vi "Ref Time series save images.vi"(8 "error in (no error)":errorcluster, 9 "Ch1-Green-REF":i16[][](graph), 10 "Ch0-Red-REF":i16[][](graph), 11 "Logging queue element":T2={"Imaging Protocol"=enum."Live Imaging", "Number of Trials"=0, "Frame Size"=512, "# Averaged frames"=0, "Dwell time (us)"=0.0, "Index of Z-plane"=0, "Timelapse?"=FALSE, "Logging process is active"=FALSE, "Speed logging enabled"=FALSE, "tdms file ref"=refnum, "path"=path "", "Trial Number"=0, "Expected # points acquired"=FALSE, "Manually stopped"=FALSE, "Last trial"=FALSE, "Ch0 data"=[], "Ch1 data"=[], "Ref Data"=[], "Ref Frame Time"=[], "Image Time"=[], "Continuous Time"=[], "Ref X Length"=0, "Ref Y Length"=0, "# Ref Averaged frames"=0, "Ref Dwell time (us)"=0.0, "Points acquired"={"Ch0 last trial"=0, "Ch1 last trial"=0, "All trials"=0}, "HW Timings File"=refnum} {"Ref Dwell time (us)" format="%#.6g"; "Frame Size" items=["100X100"=100, "128X128"=128, "200X200"=200, "256X256"=256, "512X512"=512, "1024x1024"=1024, "2048x2048"=2048]; "Dwell time (us)" format="%#.6g"}) -> (0 "error":errorcluster)   [LabVIEW 2020]
uses:
  Typedefs/Logging queue element.ctl
  Typedefs/Imaging Protocols enum.ctl
  Typedefs/Frame Size.ctl
  Typedefs/Acquired points count.ctl
  Typedefs/Channel Selector.ctl
  Typedefs/Read Write Enum.ctl
  Global Variables/General Globals.vi
panel:
  out "Imaging Protocol":T1
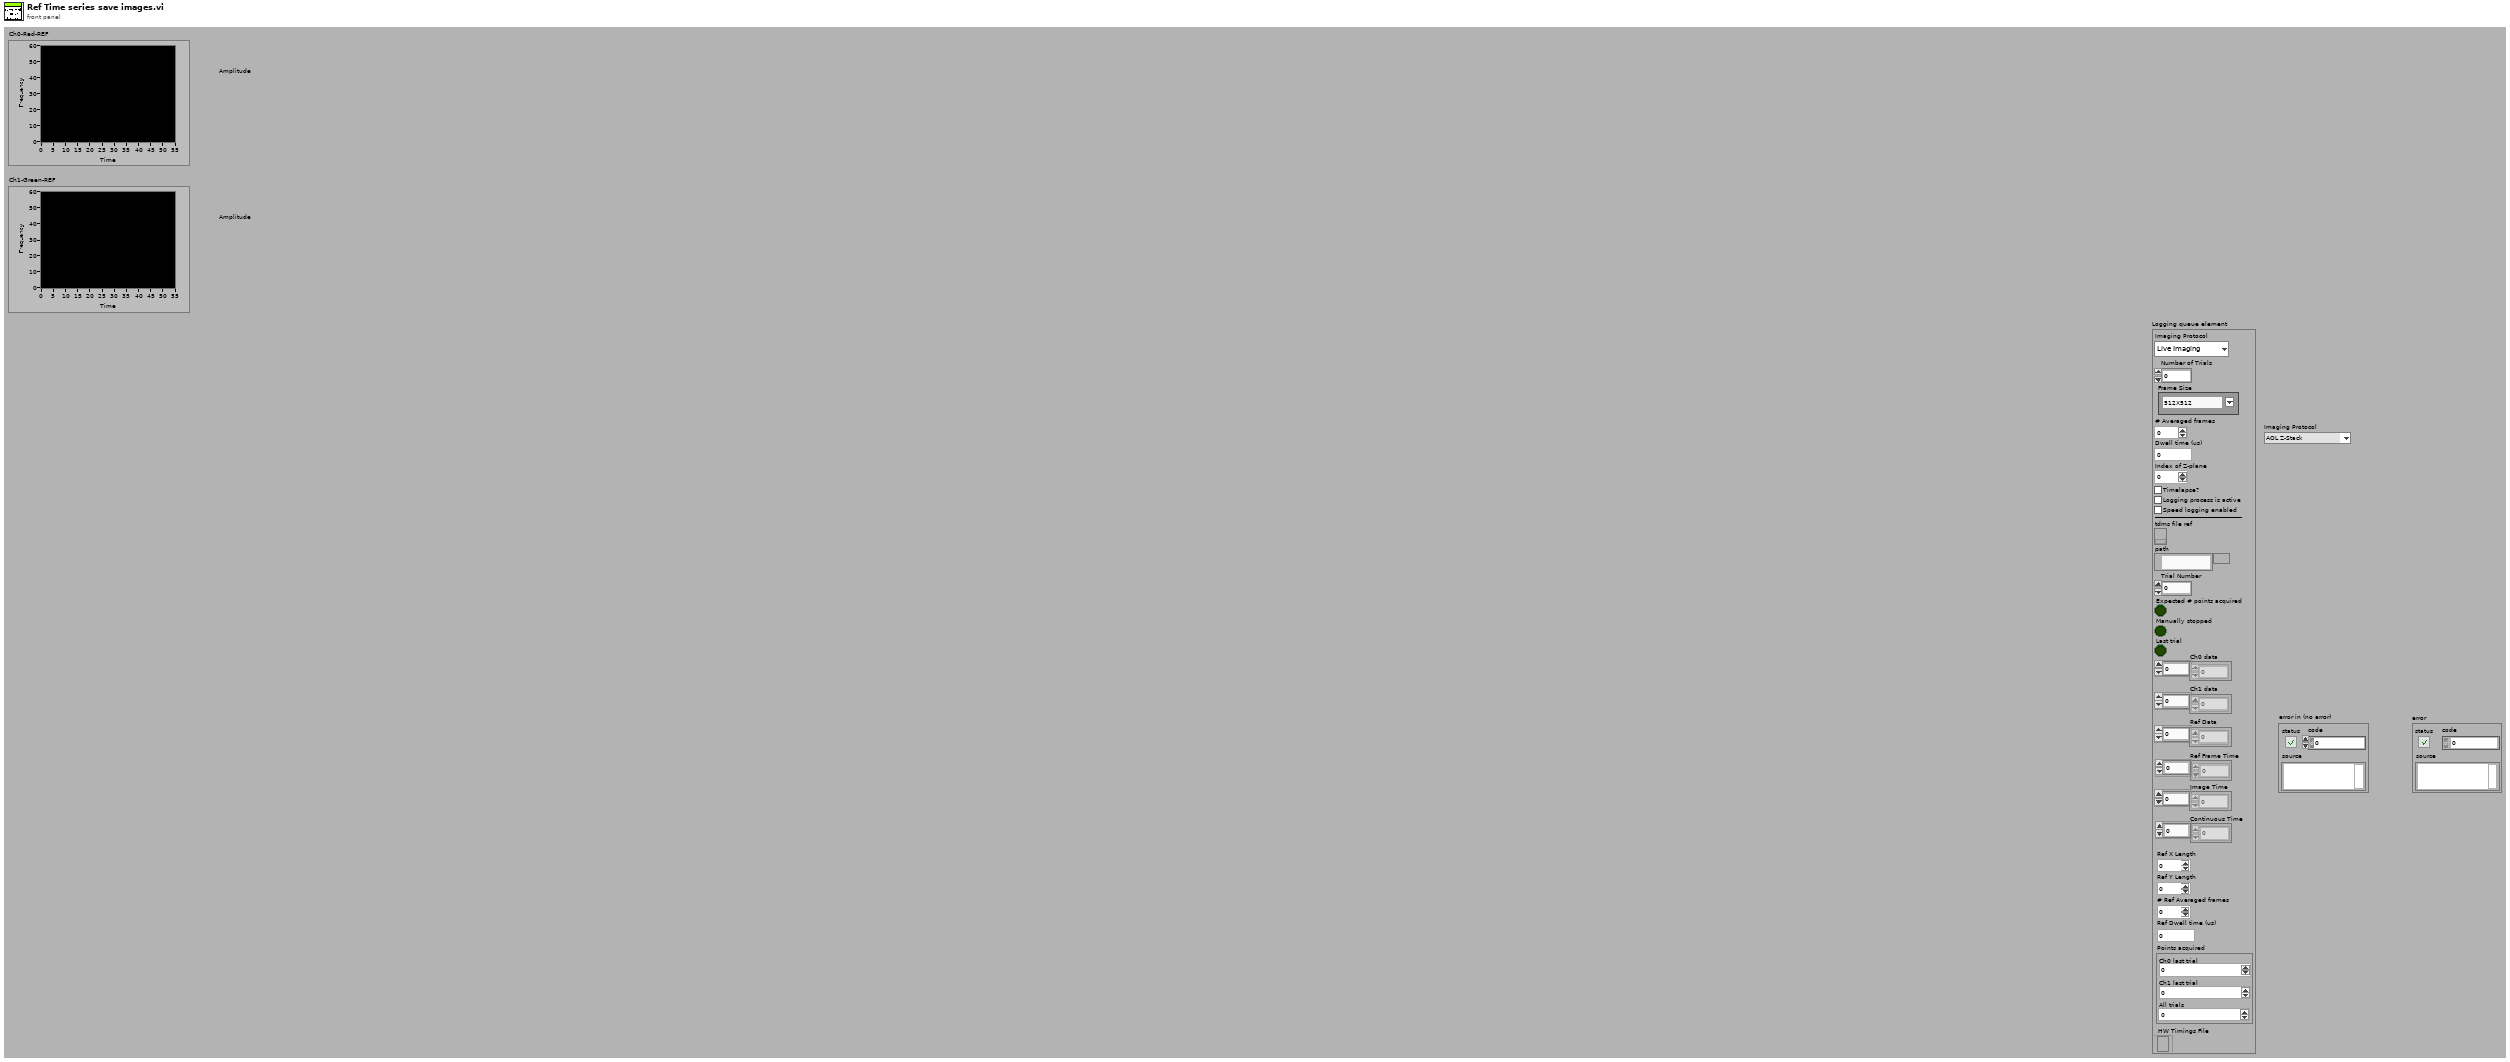
[diagram p1: front panel]
types:
  T1 = typedef "Imaging Protocols enum.ctl" = enum16{"AOL Z-Stack", "Motor Z Stack", "Functional Acquisition", "Single Plane Acquisition", "Volume Acquisition", "Live Imaging", "Live Plane Imaging", "Live Volume Imaging"}
  T2 = typedef "Logging queue element.ctl" = cluster{"Imaging Protocol":T1, "Number of Trials":u16, "Frame Size":T3, "# Averaged frames":u16, "Dwell time (us)":dbl, "Index of Z-plane":i32, "Timelapse?":bool, "Logging process is active":bool, "Speed logging enabled":bool, "tdms file ref":refnum<k34>, "path":path, "Trial Number":i32, "Expected # points acquired":bool, "Manually stopped":bool, "Last trial":bool, "Ch0 data":u32[], "Ch1 data":u32[], "Ref Data":u32[], "Ref Frame Time":u64[], "Image Time":u64[], "Continuous Time":u64[], "Ref X Length":u16, "Ref Y Length":u16, "# Ref Averaged frames":u16, "Ref Dwell time (us)":dbl, "Points acquired":T4, "HW Timings File":refnum<file>}
  T3 = typedef "Frame Size.ctl" = u16
  T4 = typedef "Acquired points count.ctl" = cluster{"Ch0 last trial":u64, "Ch1 last trial":u64, "All trials":u64}
  T5 = typedef "Channel Selector.ctl" = enum16{"Red Channel", "Green Channel", "Blended"}
  T6 = typedef "Read Write Enum.ctl" = enum16{"Read", "Write"}
  T7 = typedef "AVI implementation enum.ctl" = enum16{"AVI1", "AVI2"}
  T8 = typedef "AVI Refs cluster.ctl" = cluster{"AVI2 path":path, "AVI 2 Refnum":T9, "New Image":T10, "error out":errorcluster, "Avi 1 Refnum":T11}
  T9 = typedef "IMAQ AVI2 Refnum.ctl" = refnum<k20>
  T10 = typedef "IMAQ Image.ctl" = refnum<image>
  T11 = typedef "AviRefnum.ctl" = refnum<k1>
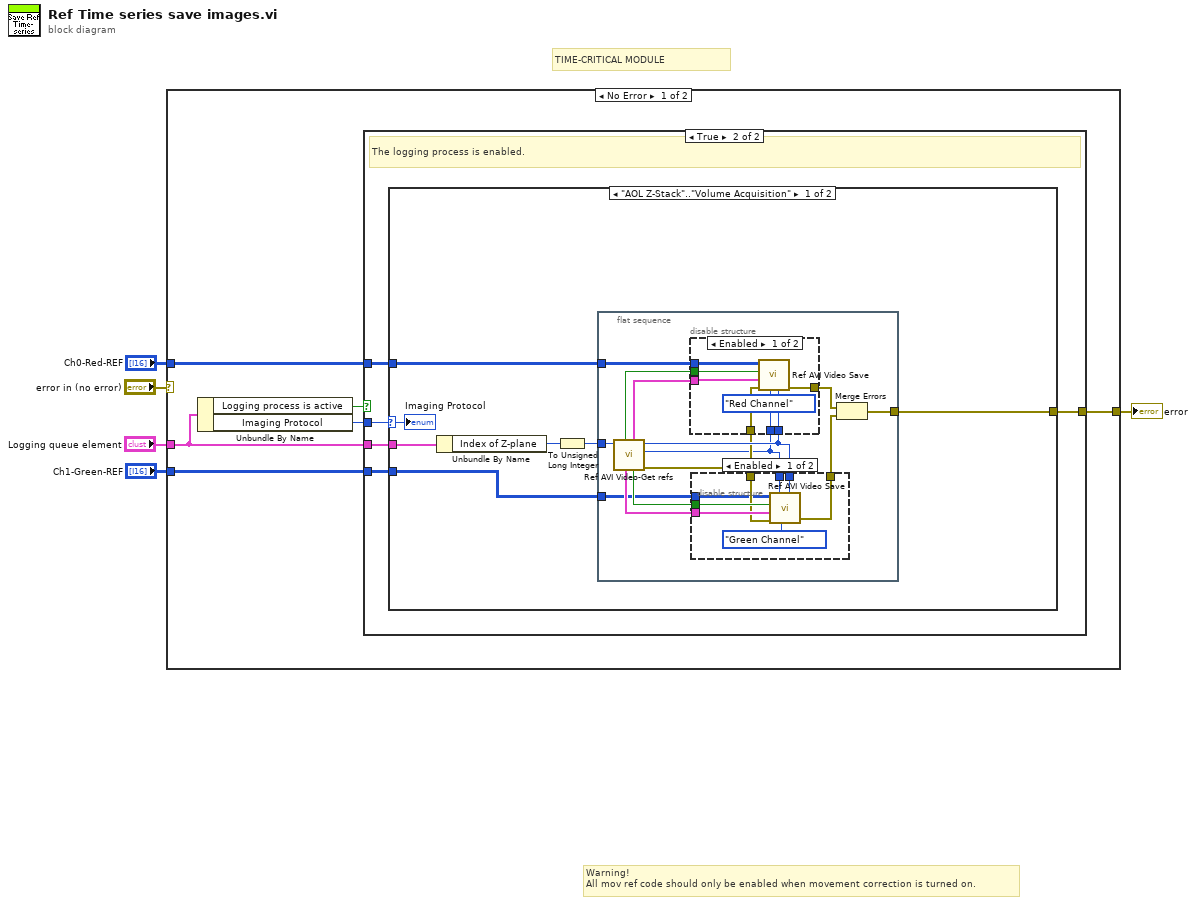
[diagram p0: block diagram]
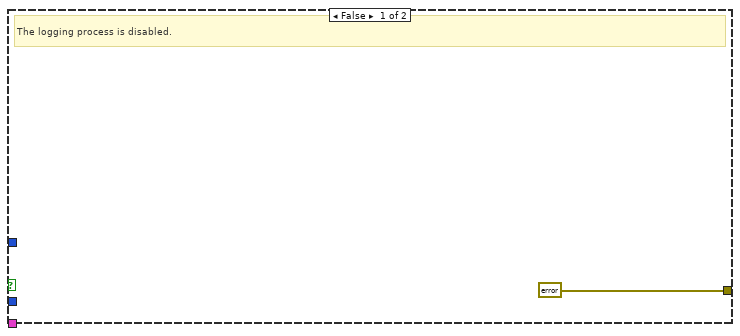
[diagram p2: hidden frame]
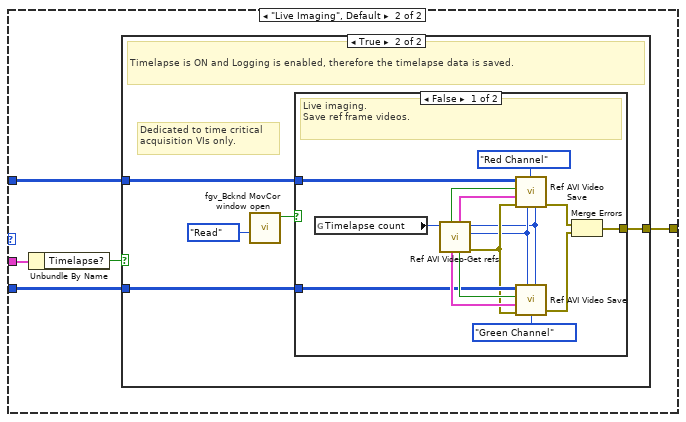
[diagram p5: hidden frame]
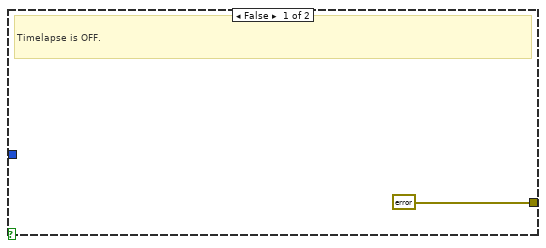
[diagram p6: hidden frame]
diagram:
  # "TIME-CRITICAL MODULE"
  # "Warning!\nAll mov ref code should only be enabled when movement correction is turned on."
  n1 = case shown="No Error" "error in (no error)" {
    selector: "error in (no error)" -> [_ w81]
    tunnel: [w11 w81] -> w5
    tunnel: "Logging queue element" -> [w6 _]
    tunnel: "Ch1-Green-REF" -> [w9 _]
    tunnel: "Ch0-Red-REF" -> [w8 _]
    frame No Error {
      n2 = Unbundle By Name(w6) -> ("Logging process is active"=w10:bool, "Imaging Protocol"=w7:T1)
      n3 = case shown="True" w10 {
        tunnel: [errorcluster {"status"=FALSE, "code"=0, "source"=""} ("error IO") w17] -> w11
        tunnel: w9 -> [_ w16]
        tunnel: w8 -> [_ w15]
        tunnel: w7 -> [_ w14]
        tunnel: w6 -> [_ w13]
        frame False {
          # "The logging process is disabled."
        }
        frame True {
          # "The logging process is enabled."
          n4 = case shown="\"AOL Z-Stack\"..\"Volume Acquisition\"" w14 {
            selector: w14 -> [w18 _]
            tunnel: [w22 w59] -> w17
            tunnel: w16 -> [w24 w58]
            tunnel: w15 -> [w23 w57]
            tunnel: w13 -> [w20 w55]
            frame "AOL Z-Stack".."Volume Acquisition" {
              n5 = Unbundle By Name(w20) -> ("Index of Z-plane"=w21:i32)
              n6 = To Unsigned Long Integer(number=w21) -> (unsigned 32bit integer=w19:u32)
              n7 = flat-sequence {
                tunnel: w24 -> [w29]
                tunnel: w23 -> [w28]
                tunnel: [w27] -> w22
                tunnel: w19 -> [w25]
                frame #0 {
                  n8 = call "Ref AVI Video-Get refs.vi"("Timelapse count"=w25) -> ("error out"=w30:errorcluster, "AVI mode"=w26:T7, "Ref X Length"=w32:u32, "Green PMT is ON"=w36:bool, "Red AVI"=w33:T8, "Green AVI"=w37:T8, "Red PMT is ON"=w31:bool)  [unwired: 3 in, 1 out]
                  n9 = disable-structure shown="Enabled" {
                    disable-tunnel: w28 -> [w52 _]
                    disable-tunnel: [w51 w54] -> w34
                    disable-tunnel: w33 -> [w50 _]
                    disable-tunnel: w26 -> [w49 _]
                    disable-tunnel: w32 -> [w48 _]
                    disable-tunnel: w31 -> [w47 _]
                    disable-tunnel: w30 -> [w46 w54]
                    frame Enabled {
                      n10 = call "Ref AVI Video Save.vi"("Frame Size"=w48, "Channel"=Channel_Selector."Red Channel", "AVI mode"=w49, "error in (no error)"=w46, "AVI cluster"=w50, "PMT is ON?"=w47, "Image Pixels"=w52) -> ("error out"=w51:errorcluster)  [unwired: 3 in, 1 out]
                    }
                    frame Disabled {
                    }
                  }
                  n11 = disable-structure shown="Enabled" {
                    disable-tunnel: w37 -> [w45 _]
                    disable-tunnel: w36 -> [w43 _]
                    disable-tunnel: [w42 _] -> w35
                    disable-tunnel: w32 -> [w41 _]
                    disable-tunnel: w30 -> [w40 _]
                    disable-tunnel: w29 -> [w39 _]
                    disable-tunnel: w26 -> [w38 _]
                    frame Enabled {
                      n12 = call "Ref AVI Video Save.vi"("Frame Size"=w41, "Channel"=Channel_Selector."Green Channel", "AVI mode"=w38, "error in (no error)"=w40, "AVI cluster"=w45, "PMT is ON?"=w43, "Image Pixels"=w39) -> ("error out"=w42:errorcluster)  [unwired: 3 in, 1 out]
                    }
                    frame Disabled {
                    }
                  }
                  n13 = Merge Errors(w34, w35) -> (w27:errorcluster)
                }
              }
              "Imaging Protocol" <- w18
            }
            frame "Live Imaging", Default {
              n14 = Unbundle By Name(w55) -> ("Timelapse?"=w56:bool)
              n15 = case shown="True" w56 {
                tunnel: [errorcluster {"status"=FALSE, "code"=0, "source"=""} ("error IO") w65] -> w59
                tunnel: w58 -> [_ w64]
                tunnel: w57 -> [_ w63]
                frame False {
                  # "Timelapse is OFF."
                }
                frame True {
                  # "Dedicated to time critical acquisition VIs only."
                  # "Timelapse is ON and Logging is enabled, therefore the timelapse data is saved."
                  n16 = call "fgv_Bcknd MovCor window open.vi"("Function"=Read_Write_Enum."Read") -> ("Background MovCor window is open"=w61:bool)  [unwired: 9 in, 1 out]
                  n17 = case shown="False" w61 {
                    tunnel: [w80 _] -> w65
                    tunnel: w64 -> [w73 _]
                    tunnel: w63 -> [w72 _]
                    frame False {
                      # "Live imaging.\nSave ref frame videos."
                      n18 = global read "General Globals.vi" "Timelapse count"() -> (w67:u32)
                      n19 = call "Ref AVI Video-Get refs.vi"("Timelapse count"=w67) -> ("error out"=w71:errorcluster, "AVI mode"=w70:T7, "Ref X Length"=w69:u32, "Green PMT is ON"=w77:bool, "Red AVI"=w75:T8, "Green AVI"=w79:T8, "Red PMT is ON"=w74:bool)  [unwired: 3 in, 1 out]
                      n20 = call "Ref AVI Video Save.vi"("Frame Size"=w69, "Channel"=Channel_Selector."Red Channel", "AVI mode"=w70, "error in (no error)"=w71, "AVI cluster"=w75, "PMT is ON?"=w74, "Image Pixels"=w72) -> ("error out"=w76:errorcluster)  [unwired: 3 in, 1 out]
                      n21 = call "Ref AVI Video Save.vi"("Frame Size"=w69, "Channel"=Channel_Selector."Green Channel", "AVI mode"=w70, "error in (no error)"=w71, "AVI cluster"=w79, "PMT is ON?"=w77, "Image Pixels"=w73) -> ("error out"=w68:errorcluster)  [unwired: 3 in, 1 out]
                      n22 = Merge Errors(w76, w68) -> (w80:errorcluster)
                    }
                    frame True {
                      # "Backgroung MovCor imaging.\nDo not save ref frame videos."
                    }
                  }
                }
              }
            }
          }
        }
      }
    }
    frame Error {
    }
  }
  "error" <- w5
